vi "TextToBorderRect.vi"(10 "Border Thickness":i16=1, 11 "Text Rect":T1) -> (3 "Border Rect":T1)   [LabVIEW 2020, in "NI_XNodeSupport.lvlib"]
uses:
  NI_XNodeSupport.lvlib
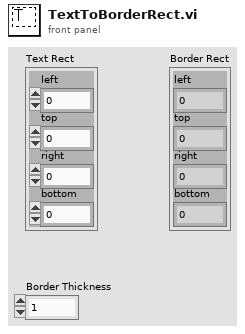
[diagram p1: front panel]
types:
  T1 = cluster{"left":i16, "top":i16, "right":i16, "bottom":i16}
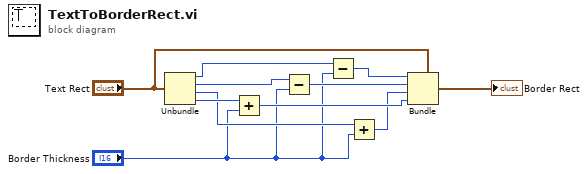
[diagram p0: block diagram]
diagram:
  n1 = Unbundle("Text Rect") -> ("left"=w5:i16, "top"=w9:i16, "right"=w2:i16, "bottom"=w8:i16)
  n2 = Add(x=w8, y="Border Thickness") -> (x+y=w7:i16)
  n3 = Subtract(x=w9, y="Border Thickness") -> (x-y=w6:i16)
  n4 = Subtract(x=w5, y="Border Thickness") -> (x-y=w4:i16)
  n5 = Add(x=w2, y="Border Thickness") -> (x+y=w3:i16)
  n6 = Bundle(cluster="Text Rect", "left"=w4, "top"=w6, "right"=w3, "bottom"=w7) -> (→"Border Rect":T1)
